vi "(SubVI)_Imp_tab_IO_Initialization.vi"(6 "Data Array [Sti.Gal.AO0; sti.Gal.AO1; Laser driver AO2]":dbl[][](array[numeric]) format="%0.2f", 7 "Sti. Gal and Laser Driver 3 AOs Ctr Term (PFI2)":tag="/Dev5/PFI2", 8 "Sti. Gal and Laser Driver 3 AOs Ctr (Ctr2)":tag="Dev5/ctr2", 9 "Sti. Galvo AO(0:1) and Laser Driver AO(2) Chns":tag="Dev5/ao0:2") -> (0 "error out Ini of IO Chs":errorcluster, 2 "Sti. Gal and Laser Driver 3 AOs Ctr Task Out":refnum<k21>, 3 "Sti. Galvo AOs and Laser Driver AO Task Out":refnum<k21>)   [LabVIEW 2019]
uses:
  <vilib>/DAQmx/write.llb/DAQmx Write (Analog 2D DBL NChan NSamp).vi
  <vilib>/DAQmx/create/channels.llb/DAQmx Create Channel (AO-Voltage-Basic).vi
  <vilib>/DAQmx/configure/timing.llb/DAQmx Timing (Sample Clock).vi
  <vilib>/DAQmx/miscellaneous.llb/DAQmx Fill In Error Info.vi
  <vilib>/DAQmx/create/channels.llb/DAQmx Create Channel (CO-Pulse Generation-Frequency).vi
  <vilib>/DAQmx/configure/timing.llb/DAQmx Timing (Implicit).vi
  <resource>/objmgr/daqmx.rc
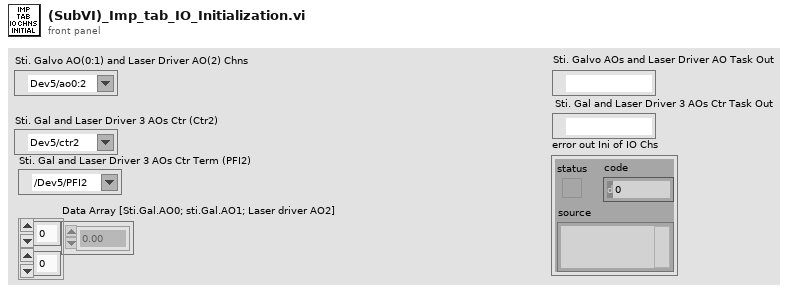
[diagram p1: front panel]
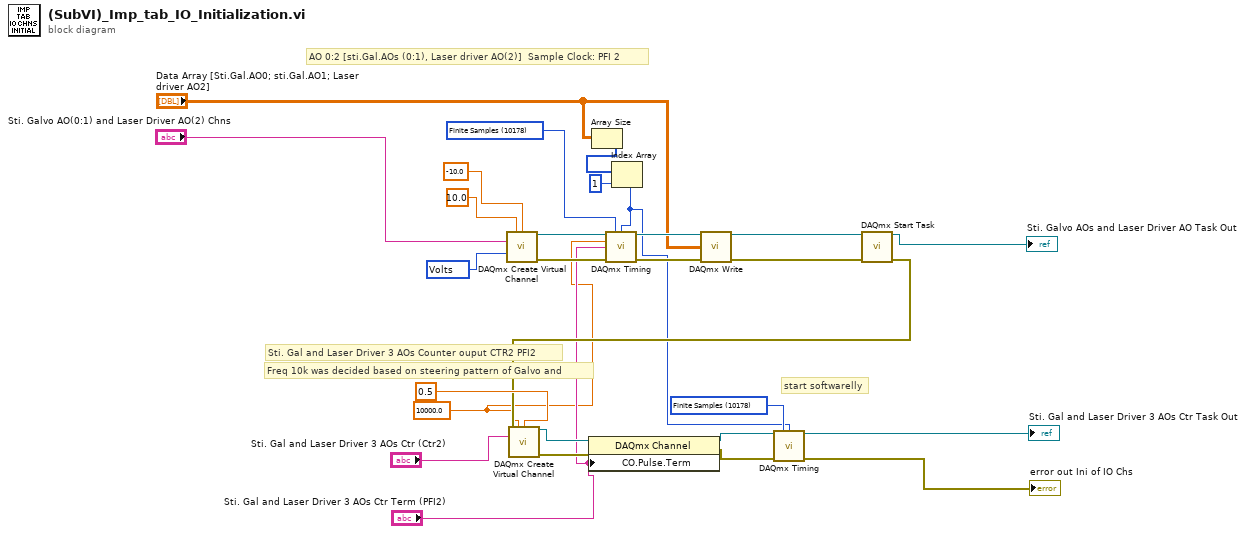
[diagram p0: block diagram]
diagram:
  w10 = 10178 items=["Finite Samples"=10178, "Continuous Samples"=10123, "Hardware Timed Single Point"=12522] ("sample mode")
  w1 = 10000.0 ("frequency")
  w25 = 10348 items=["Volts"=10348, "From Custom Scale"=10065] ("units")
  w21 = 10178 items=["Finite Samples"=10178, "Continuous Samples"=10123] ("sample mode")
  # "Freq 10k was decided based on steering pattern of Galvo and"
  # "start softwarelly"
  # "Sti. Gal and Laser Driver 3 AOs Counter ouput CTR2 PFI2"
  # "AO 0:2 [sti.Gal.AOs (0:1), Laser driver AO(2)]  Sample Clock: PFI 2"
  n1 = call-poly <vilib>:"DAQmx Create Virtual Channel.vi"("maximum value"=10.0, "minimum value"=-10.0, "physical channels"="Sti. Galvo AO(0:1) and Laser Driver AO(2) Chns", "units"=w25) -> ("task out"=w2:refnum<k21>, "error out"=w26:errorcluster)  [unwired: 5 in, 5 out]
  n2 = Array Size(array="Data Array [Sti.Gal.AO0; sti.Gal.AO1; Laser driver AO2]") -> (size(s)=w14:i32[])
  n3 = Index Array(array=w14, index=1) -> (element=w9:i32)
  n4 = call-poly <vilib>:"DAQmx Timing.vi"("task/channels in"=w2, "sample mode"=w21, "samples per channel"=w9, "rate"=w1, "source"="Sti. Gal and Laser Driver 3 AOs Ctr Term (PFI2)", "error in"=w26) -> ("task out"=w27:refnum<k21>, "error out"=w28:errorcluster)  [unwired: 8 in]
  n5 = call-poly <vilib>:"DAQmx Write.vi"("task/channels in"=w27, "data"="Data Array [Sti.Gal.AO0; sti.Gal.AO1; Laser driver AO2]", "error in"=w28) -> ("task out"=w6:refnum<k21>, "error out"=w5:errorcluster)  [unwired: 1 in, 10 out]
  n6 = call <vilib>:"DAQmx Start Task.vi"("task/channels in"=w6, "error in"=w5) -> ("task out"=→"Sti. Galvo AOs and Laser Driver AO Task Out":refnum<k21>, "error out"=w18:errorcluster)  [unwired: 12 in]
  n7 = call-poly <vilib>:"DAQmx Create Virtual Channel.vi"("frequency"=w1, "duty cycle"=0.5, "counter"="Sti. Gal and Laser Driver 3 AOs Ctr (Ctr2)", "error in"=w18) -> ("task out"=w17:refnum<k21>, "error out"=w16:errorcluster)  [unwired: 5 in, 5 out]
  n8 = property class="DAQmx Channel"(reference=w17, error in=w16, "CO.Pulse.Term"="Sti. Gal and Laser Driver 3 AOs Ctr Term (PFI2)") -> (reference out=w12:refnum<k21>, error out=w11:errorcluster)
  n9 = call-poly <vilib>:"DAQmx Timing.vi"("task/channels in"=w12, "sample mode"=w10, "samples per channel"=w9, "error in"=w11) -> ("task out"=→"Sti. Gal and Laser Driver 3 AOs Ctr Task Out":refnum<k21>, "error out"=→"error out Ini of IO Chs":errorcluster)  [unwired: 10 in]
